vi "rethinkdb_msg_auth_client_first.vi"(8 "error in (no error)":errorcluster, 10 "password":string, 11 "user":string) -> (0 "error out":errorcluster, 2 "client hash":u32[](array[numeric]) format="%08x", 3 "auth client first":string)   [LabVIEW 2017]
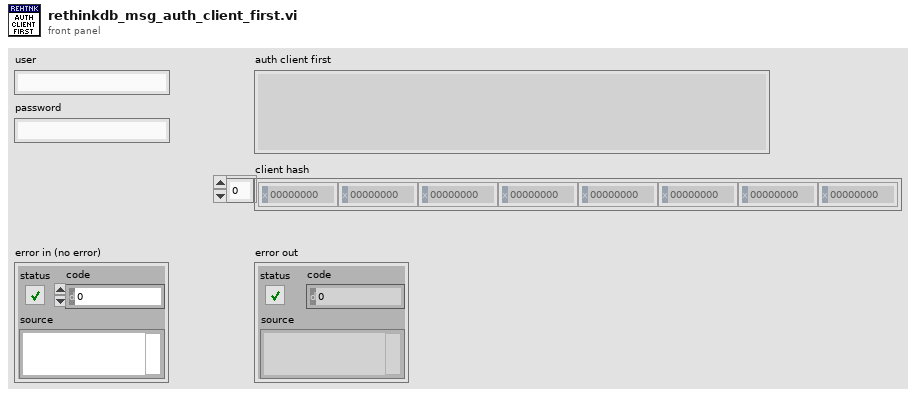
[diagram p1: front panel]
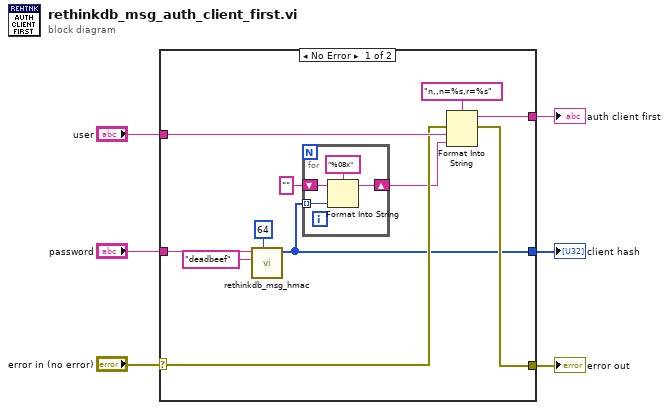
[diagram p0: block diagram]
diagram:
  n1 = case shown="No Error" "error in (no error)" {
    selector: "error in (no error)" -> [w13 w22]
    tunnel: "password" -> [w11 _]
    tunnel: "user" -> [w16 _]
    tunnel: [w15 w22] -> w3
    tunnel: [w14 _] -> w2
    tunnel: [w10 _] -> w1
    frame No Error {
      n2 = call "rethinkdb_msg_hmac.vi"("blocksize (SHA256=64)"=64, "message"="deadbeef", "key"=w11) -> ("sha-256 hash"=w10:u32[])  [unwired: 8 in]
      n3 = for {
        tunnel: w10 -> [w20] mode=indexing
        shift-right: [w19] -> w7
        shift-left: "" -> [w18]
        n4 = Format Into String(format string="%08x", initial string=w18, w20) -> (resulting string=w19:string)  [unwired: 1 in, 1 out]
      }
      n5 = Format Into String(format string="n,,n=%s,r=%s" ("auth client first"), error in=w13, w16, w7) -> (resulting string=w14:string, error out=w15:errorcluster)  [unwired: 1 in]
    }
    frame Error {
    }
  }
  "error out" <- w3
  "auth client first" <- w2
  "client hash" <- w1
